vi "Read predef by index.vi"(8 "error in (no error)":errorcluster, 10 "index":string, 11 "Motor in":refnum<class "Motor.lvclass">) -> (0 "error out":errorcluster, 1 "pos_name":string, 2 "pos_value":string, 3 "Motor out":refnum<class "Motor.lvclass">)   [LabVIEW 2018, in "Motor.lvclass"]
uses:
  Motor.lvclass
  Motor.lvclass/Motor.ctl
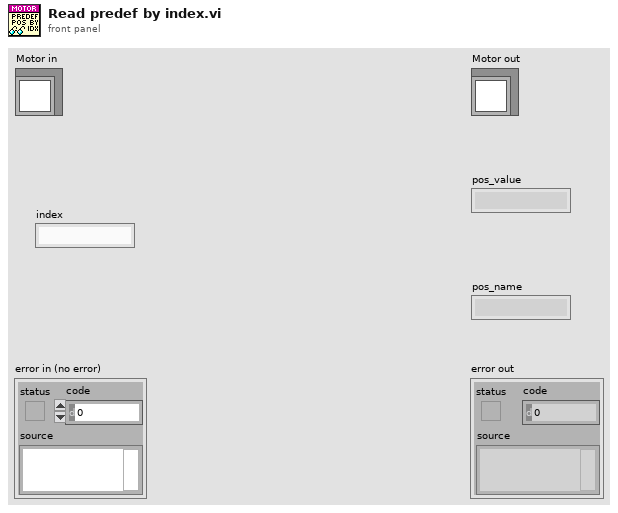
[diagram p1: front panel]
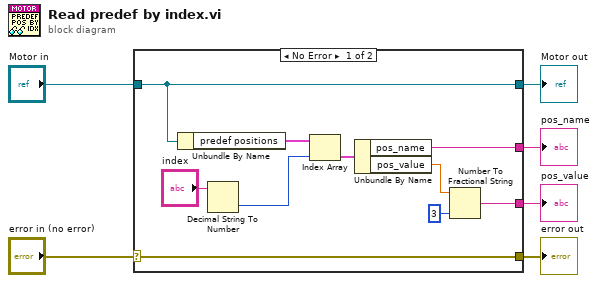
[diagram p0: block diagram]
diagram:
  n1 = case shown="No Error" "error in (no error)" {
    selector: "error in (no error)" -> [w16 w17]
    tunnel: [w16 w17] -> w5
    tunnel: [w15 w18] -> w3
    tunnel: "Motor in" -> [w15 w18]
    tunnel: [w12 _] -> w2
    tunnel: [w7 _] -> w1
    frame No Error {
      n2 = Unbundle By Name(w15) -> ("predef positions"=w14:cluster{"pos_name":string, "pos_value":dbl}[])
      n3 = Decimal String To Number(string="index") -> (number=w11:i32)  [unwired: 2 in, 1 out]
      n4 = Index Array(array=w14, index=w11) -> (element=w13:cluster{"pos_name":string, "pos_value":dbl})
      n5 = Unbundle By Name(w13) -> ("pos_name"=w12:string, "pos_value"=w9:dbl)
      n6 = Number To Fractional String(number=w9, precision (6)=i16 3) -> (F-format string=w7:string)  [unwired: 2 in]
    }
    frame Error {
    }
  }
  "error out" <- w5
  "Motor out" <- w3
  "pos_name" <- w2
  "pos_value" <- w1
